vi "Get Register Address Field Width.vi"(8 "error in (no error)":errorcluster, 11 "RFFE Standard Command in":refnum<class "RFFE Standard Command.lvclass">) -> (0 "error out":errorcluster, 2 "Register Address Field Width":i32, 3 "RFFE Standard Command out":refnum<class "RFFE Standard Command.lvclass">)   [LabVIEW 2018, in "MIPI RFFE API.lvlib" / "RFFE Standard Command.lvclass"]
uses:
  RFFE Standard Command.lvclass
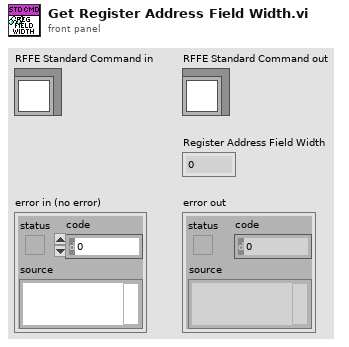
[diagram p1: front panel]
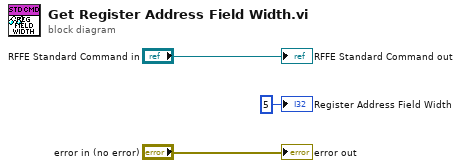
[diagram p0: block diagram]
diagram:
  "error out" <- "error in (no error)"
  "RFFE Standard Command out" <- "RFFE Standard Command in"
  "Register Address Field Width" <- 5 ("Register Address Field Width")
